vi "Build_Asylum_StopInWaveBank.vi"(8 "error in (no error)":errorcluster, 11 "whichBank":i32) -> (0 "error out":errorcluster, 3 "Command":string)   [LabVIEW 2019]
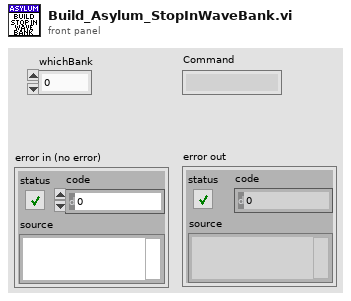
[diagram p1: front panel]
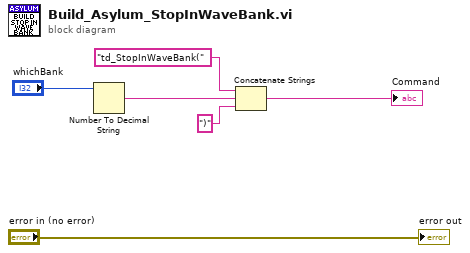
[diagram p0: block diagram]
diagram:
  n1 = Number To Decimal String(number="whichBank") -> (decimal integer string=w3:string)  [unwired: 1 in]
  n2 = Concatenate Strings("td_StopInWaveBank(" ("string"), w3, ")" ("string")) -> (→"Command":string)
  "error out" <- "error in (no error)"
